vi "post_dcs_spot.vi"(8 "error in (no error)":errorcluster, 11 "dcs_spot":T1={"DCS spot ID"=0, "Integer Timestamp"=2, "Spot X"=3.0, "Spot Y"=4.0, "Spot Width X"=0.0, "Spot Width Y"=0.0, "Spot Size"=0, "Experiment Settings ID"=0}) -> (0 "error out":errorcluster)   [LabVIEW 2013]
doc: "Adds a new row to the dcs_spot table."
uses:
  User Interface/Controls/dcs_spot.ctl
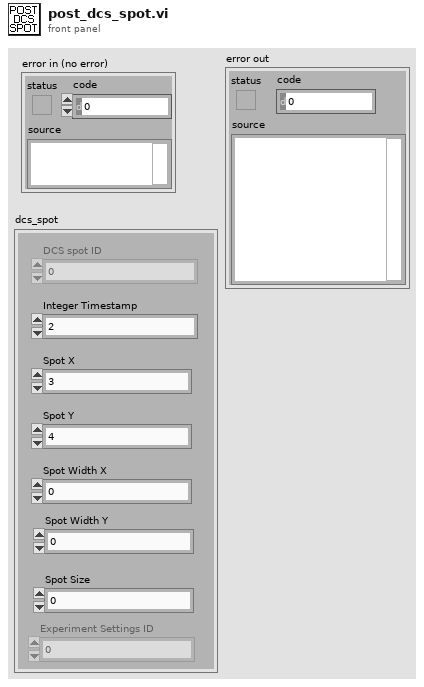
[diagram p1: front panel]
types:
  T1 = typedef "dcs_spot.ctl" = cluster{"DCS spot ID":i32, "Integer Timestamp":i64, "Spot X":dbl, "Spot Y":dbl, "Spot Width X":dbl, "Spot Width Y":dbl, "Spot Size":i32, "Experiment Settings ID":i32}
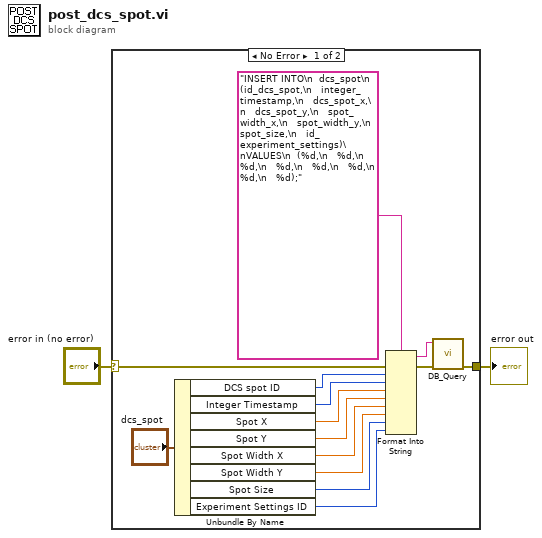
[diagram p0: block diagram]
diagram:
  n1 = case shown="No Error" "error in (no error)" {
    selector: "error in (no error)" -> [w15 w17]
    tunnel: [w3 w17] -> w1
    frame No Error {
      n2 = Unbundle By Name("dcs_spot") -> ("DCS spot ID"=w12:i32, "Integer Timestamp"=w11:i64, "Spot X"=w10:dbl, "Spot Y"=w9:dbl, "Spot Width X"=w8:dbl, "Spot Width Y"=w7:dbl, "Spot Size"=w6:i32, "Experiment Settings ID"=w5:i32)
      n3 = Format Into String(format string="INSERT INTO\n  dcs_spot\n  (id_dcs_spot,\n   integer_timestamp,\n   dcs_spot_x,\n   dcs_spot_y,\n   spot_width_x,\n   spot_width_y,\n   spot_size,\n   id_experiment_settings)\nVALUES\n  (%d,\n   %d,\n   %d,\n   %d,\n   %d,\n   %d,\n   %d,\n   %d);" ("Parameterized Query"), error in=w15, w12, w11, w10, w9, w8, w7, w6, w5) -> (resulting string=w4:string, error out=w14:errorcluster)  [unwired: 1 in]
      n4 = call "DB_Query.vi"("error in (no error)"=w14, "Parameterized Query"=w4) -> ("error out"=w3:errorcluster)  [unwired: 7 in, 2 out]
    }
    frame Error {
    }
  }
  "error out" <- w1
